vi "SETAGAdll.vi"(8 "error in (no error)":errorcluster) -> (0 "error out":errorcluster, 2 "herr out":string, 3 "ierr out":i32)   [LabVIEW 2016]
doc: "subroutine SETAGA (ierr,herr, herr_length)\n\nset up working arrays for use with AGA8 equation of state\n\nOUTPUTS:\nierr--error flag: 0 = successful\n 1 = error (e.g. fluid not found)\nherr--error string (character*255 variable if ierr<>0)\n [fluid parameters, etc. returned via various common blocks]\nherr_length -- length of variable herr (default: 255)"
uses:
  REFPROP.DLL
panel:
  out "herr_length":i32
  # "REFPROP-SETAGAdll.vi"
  # "void  SETAGAdll(int32_t *ierr, CStr herr, int32_t herr_length);"
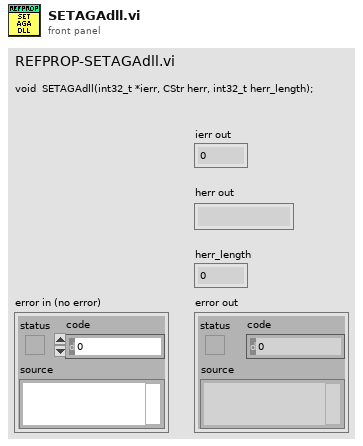
[diagram p1: front panel]
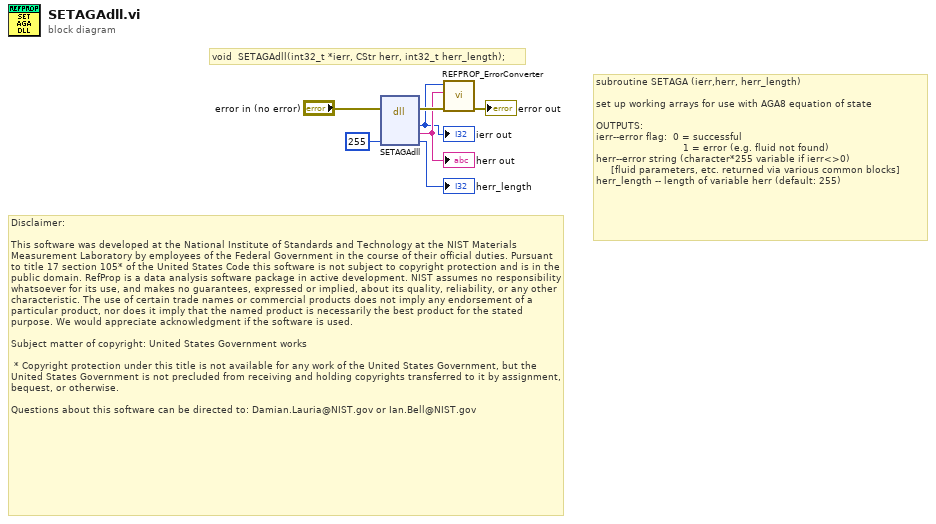
[diagram p0: block diagram]
diagram:
  # "Disclaimer:\n\nThis software was developed at the National Institute of Standards and Technology at the NIST Materials Measurement Laboratory by employees of the Federal Government in the course of their official duties. Pursuant to title 17 section 105* of the United States Code this software is not subject to copyright protection and is in the public domain. RefProp is a data analysis software package in active development. NIST assumes no responsibility whatsoever for its use, and makes no guarantees, expressed or implied, about its quality, reliability, or any other characteristic. The use of certain trade names or commercial products does not imply any endorsement of a particular product, nor does it imply that the named product is necessarily the best product for the stated purpose. We would appreciate acknowledgment if the software is used.\n \nSubject matter of copyright: United States Government works\n  \n * Copyright protection under this title is not available for any work of the United States Government, but the United States Government is not precluded from receiving and holding copyrights transferred to it by assignment, bequest, or otherwise.\n\nQuestions about this software can be directed to: Damian.Lauria@NIST.gov or Ian.Bell@NIST.gov"
  # "void  SETAGAdll(int32_t *ierr, CStr herr, int32_t herr_length);"
  # "subroutine SETAGA (ierr,herr, herr_length)\n\nset up working arrays for use with AGA8 equation of state\n\nOUTPUTS:\nierr--error flag:  0 = successful\n                             1 = error (e.g. fluid not found)\nherr--error string (character*255 variable if ierr<>0)\n     [fluid parameters, etc. returned via various common blocks]\nherr_length -- length of variable herr (default: 255)"
  n1 = dll-call lib="S:/009 - Testing/02 - Performance Testing/REFPROP/REFPROP.*" fn="SETAGAdll"(error in="error in (no error)", "herr_length"=255) -> (error out=w7:errorcluster, "ierr"=w1:i32, "herr"=w2:string, "herr_length"=→"herr_length":i32)  [unwired: 5 in, 1 out]
  "ierr out" <- w1
  "herr out" <- w2
  n2 = call "REFPROP_ErrorConverter.vi"("error in (no error)"=w7, "Error Message"=w2, "Error Code"=w1) -> ("error out"=→"error out":errorcluster)  [unwired: 8 in]
